vi "Zero Yaw.vi"(7 "Device Number":T1, 10 "Zero":bool) -> ()   [LabVIEW 2016]
uses:
  <vilib>/Rock Robotics/WPI/ThirdParty/Sensors/navX/_TypeDefs/FRIC_navX_DeviceNumbersTypeDef.ctl
  <vilib>/Rock Robotics/WPI/ThirdParty/Sensors/navX/_TypeDefs/Z900_navX_ActionTypeDef.ctl
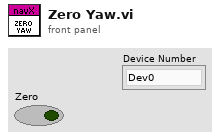
[diagram p1: front panel]
types:
  T1 = typedef "FRIC_navX_DeviceNumbersTypeDef.ctl" = enum16{"Dev0", "Dev1", "Dev2", "Dev3"}
  T2 = typedef "Z900_navX_ActionTypeDef.ctl" = enum16{"None", "Halt", "Normal Read", "Update Serial Protocol", "Update Rate Htz", "Zero-Yaw", "Zero-Displacement", "Zero-Velocity"}
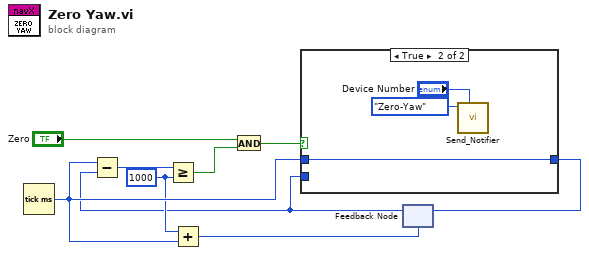
[diagram p0: block diagram]
diagram:
  w4 = u32 1000 ("y")
  n1 = Tick Count (ms)() -> (millisecond timer value=w5:u32)
  n2 = Add(x=w4, y=w5) -> (x+y=w3:u32)
  n3 = feedback #1(w3) -> (w1:u32)
  n4 = Subtract(x=w5, y=w1) -> (x-y=w6:u32)
  n5 = Greater Or Equal?(x=w6, y=w4) -> (x >= y?=w2:bool)
  n6 = And(x="Zero", y=w2) -> (x .and. y?=w8:bool)
  n7 = case shown="True" w8 {
    tunnel: [w10 w13] -> w7
    tunnel: w5 -> [_ w13]
    tunnel: w1 -> [w10 _]
    frame False {
    }
    frame True {
      n8 = call <vilib>:"Send_Notifier.vi"("Device Number"="Device Number", "navX Action"=Z900_navX_ActionTypeDef."Zero-Yaw") -> ()  [unwired: 10 in]
    }
  }
  n9 = feedback-in #1(w7) -> ()
